vi "Set Channel Value Table.vi"(8 "error in":errorcluster, 9 "values":dbl[](array[numeric]), 10 "names":string[](array[string]), 11 "channel in":T1 format="%.0x") -> (0 "error out":errorcluster, 3 "channel out":T1=18446744073709551615 format="%.0x")   [LabVIEW 2027, in "Embedded Data Logger Scripting.lvlib"]
uses:
  Embedded Data Logger Scripting.lvlib
  C:/NetCore/niveristand-embedded-data-logger-custom-device/Source/Scripting/Utility/Set Channel Value Table.vi/NationalInstruments.VeriStand.SystemDefinitionAPI
  NationalInstruments.VeriStand.SystemDefinitionAPI
  C:/NetCoreDLL/NationalInstruments.VeriStand.SystemStorage.dll
  NetCoreDLL/NationalInstruments.VeriStand.SystemStorage.dll
  <vilib>/NI VeriStand/Custom Device API/Custom Device Item Ref.ctl
  <vilib>/NI VeriStand/Custom Device API/Custom Device API.lvlib
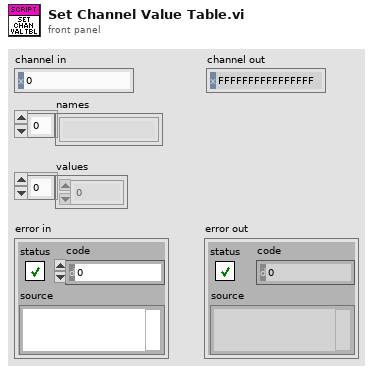
[diagram p1: front panel]
types:
  T1 = typedef "Custom Device API.lvlib/Custom Device Item Ref.ctl" = u64
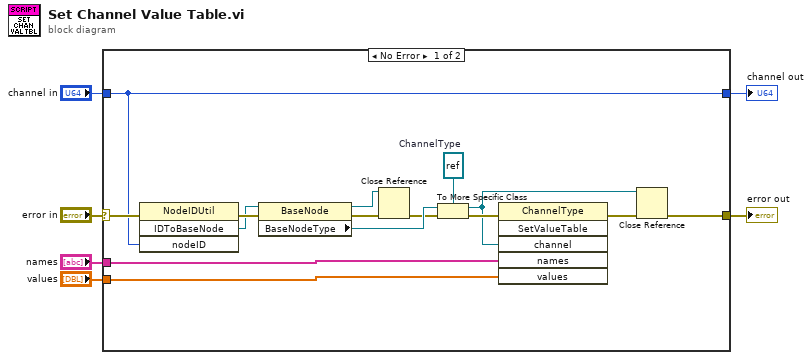
[diagram p0: block diagram]
diagram:
  n1 = case shown="No Error" "error in" {
    selector: "error in" -> [w21 w23]
    tunnel: [w20 w23] -> w6
    tunnel: "channel in" -> [w12 w22]
    tunnel: [w12 w22] -> w4
    tunnel: "names" -> [w19 _]
    tunnel: "values" -> [w18 _]
    frame No Error {
      w15 = refnum<k39> refnum  # ChannelType
      n2 = invoke class="NodeIDUtil" method="IDToBaseNode"(error in=w21, "nodeID"=w12) -> (error out=w14:errorcluster, "IDToBaseNode"=w10:refnum<k39>)  [unwired: 2 in, 2 out]
      n3 = property class="BaseNode"(reference=w10, error in=w14) -> (reference out=w7:refnum<k39>, error out=w11:errorcluster, "BaseNodeType"=w9:refnum<k39>)
      n4 = Close Reference(reference=w7, error in (no error)=w11) -> (error out=w8:errorcluster)
      n5 = To More Specific Class(target class=w15, reference=w9, error in=w8) -> (specific class reference=w13:refnum<k39>, error out=w17:errorcluster)
      n6 = invoke class="ChannelType" method="SetValueTable"(error in=w17, "channel"=w13, "names"=w19, "values"=w18) -> (error out=w16:errorcluster)  [unwired: 2 in, 5 out]
      n7 = Close Reference(reference=w13, error in (no error)=w16) -> (error out=w20:errorcluster)
    }
    frame Error {
    }
  }
  "error out" <- w6
  "channel out" <- w4
